vi "Alicat read.vi"(8 "error out 2":errorcluster, 10 "Byte array":u8[](array[numeric])=[65, 48, 48, 48, 48, 48, 13, 66, 48, 48, 48, 48, 48, 13, 67, 48, 48, 48, 48, 48, 13, 68, 48, 48, 48, 48, 48, 13, 69, 48, 48, 48, 48, 48, 13, 70, 48, 48, 48, 48, 48, 13, 71, 48, 48, 48, 48, 48, 13, 0, 0, 0, 0, 0, 0, 0, 0, 0, 0, 0, 0, 0, 0]) -> (0 "error out":errorcluster)   [LabVIEW 2011]
uses:
  <vilib>/rvi/eio/common/nirviEmuTemplateMethod_errors.vi
  <vilib>/eio/EIOMethodNode/EIOMethodNode.xnode
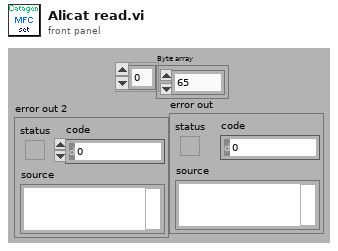
[diagram p1: front panel]
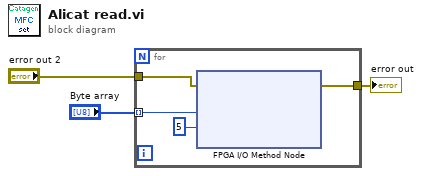
[diagram p0: block diagram]
diagram:
  n1 = for {
    tunnel: "Byte array" -> [w6] mode=indexing
    tunnel: [w5] -> w2
    tunnel: "error out 2" -> [w4]
    n2 = xnode "FPGA I/O Method Node"("error in"=w4, "Data"=w6, "Timeout (ms)"=5) -> ("error out"=w5:errorcluster)  [unwired: 1 in, 2 out]
  }
  "error out" <- w2
